vi "set_output_type.vi"(8 "error in (no error)":errorcluster, 10 "output type":T1, 11 "DAQmxWriteSignals.lvclass in":refnum<class "SignalWriterDL090202DAQmx.lvclass">) -> (0 "error out":errorcluster, 3 "DAQmxWriteSignals.lvclass out":refnum<class "SignalWriterDL090202DAQmx.lvclass">)   [LabVIEW 2010, in "SignalWriterDL090202DAQmx.lvclass"]
uses:
  SignalWriterDL090202DAQmx.lvclass
  output_type_enum.ctl
  SignalWriterDL090202DAQmx.lvclass/SignalWriterDL090202DAQmx.ctl
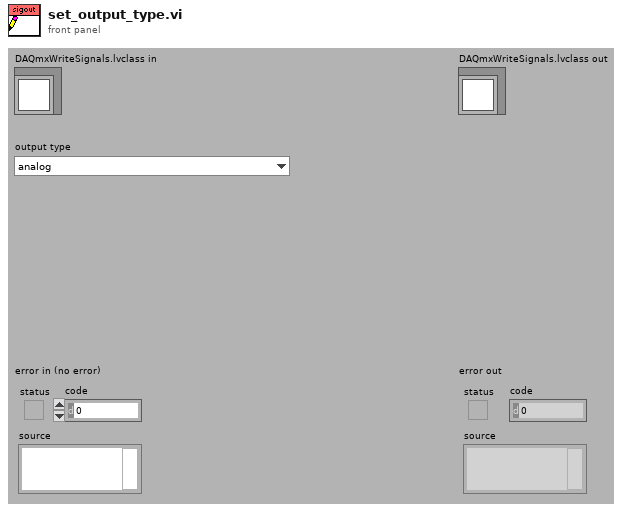
[diagram p1: front panel]
types:
  T1 = typedef "SignalWriterDL090202DAQmx.lvclass/output_type_enum.ctl" = enum16{"analog", "digital (U8)", "digital (U16)", "digital (U32)"}
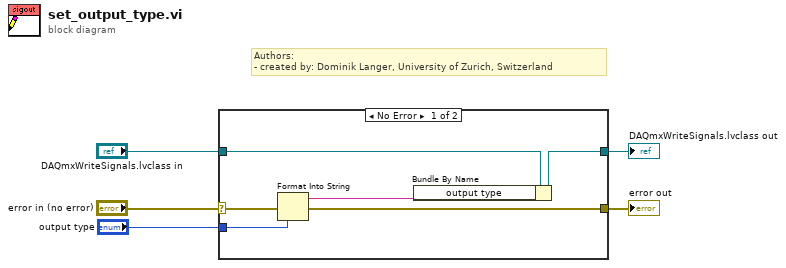
[diagram p0: block diagram]
diagram:
  # "Authors: \n- created by: Dominik Langer, University of Zurich, Switzerland"
  n1 = case shown="No Error" "error in (no error)" {
    selector: "error in (no error)" -> [w10 w12]
    tunnel: [w9 w12] -> w4
    tunnel: [w7 w13] -> w2
    tunnel: "DAQmxWriteSignals.lvclass in" -> [w8 w13]
    tunnel: "output type" -> [w11 _]
    frame No Error {
      n2 = Format Into String(error in=w10, w11) -> (resulting string=w6:string, error out=w9:errorcluster)  [unwired: 2 in]
      n3 = Bundle By Name(cluster=w8, "output type"=w6) -> (w7:refnum<class "SignalWriterDL090202DAQmx.lvclass">)
    }
    frame Error {
    }
  }
  "error out" <- w4
  "DAQmxWriteSignals.lvclass out" <- w2
